vi "Data Plot.vi"(8 "error in (no error)":errorcluster, 11 "Data DVR in":refnum<data-value>) -> (0 "error out":errorcluster, 3 "Data DVR out":refnum<data-value>)   [LabVIEW 2012, in "MDSplus.lvlib"]
doc: "Plots the data in a newly created Scope instance."
uses:
  <vilib>/MDSplus/Library/MDSplus.lvlib
  <vilib>/MDSplus/Classes/Data_Class/Data.lvclass
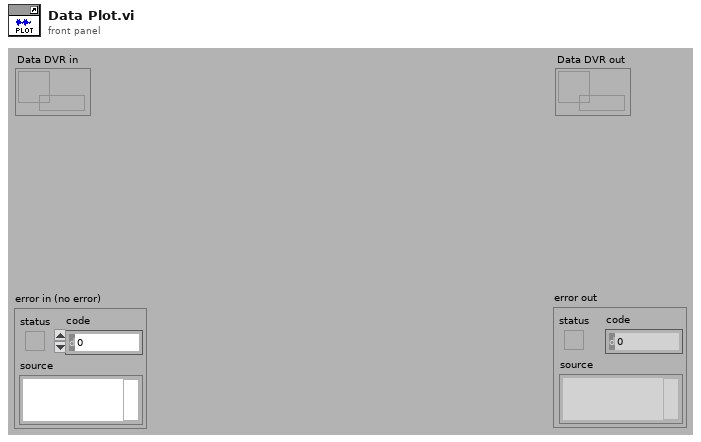
[diagram p1: front panel]
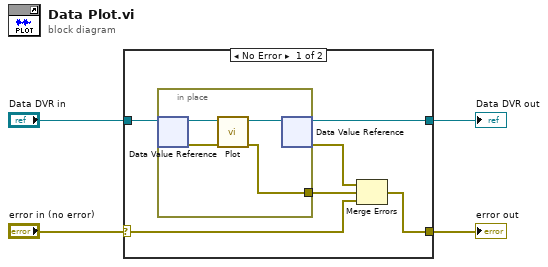
[diagram p0: block diagram]
diagram:
  n1 = case shown="No Error" "error in (no error)" {
    selector: "error in (no error)" -> [w8 w16]
    tunnel: "Data DVR in" -> [w10 w15]
    tunnel: [w7 w16] -> w4
    tunnel: [w6 w15] -> w1
    frame No Error {
      n2 = in-place {
        in-place-border: [w12] -> w9
        n3 = in-place-dvr #1(w10) -> (w14:refnum<class "Data.lvclass">, w11:errorcluster)
        n4 = call-dynamic "Plot.vi"("error in (no error)"=w11, "Data in"=w14) -> ("error out"=w12:errorcluster, "Data out"=w13:refnum<class "Data.lvclass">)  [unwired: 8 in]
        n5 = in-place-dvr #1(w13) -> (w6:refnum<data-value>, w5:errorcluster)
      }
      n6 = Merge Errors(w5, w9, w8) -> (w7:errorcluster)
    }
    frame Error {
    }
  }
  "error out" <- w4
  "Data DVR out" <- w1
